vi "Send Message.vi"(6 "priority":i32, 8 "error in (no error)":errorcluster, 9 "timeout ms (-1)":i32=-1, 10 "Message":refnum<class "Message.lvclass">, 11 "Network Stream in":refnum<class "Network Stream.lvclass">) -> (0 "error out":errorcluster, 3 "Network Stream out":refnum<class "Network Stream.lvclass">)   [LabVIEW 2023, in "Network Stream.lvclass"]
uses:
  Network Stream.lvclass
  C:/Program Files/National Instruments/LabVIEW 2023/vi.lib/ni/Actors/Network Endpoint Actors/Abstract Classes/Message Stream/Message Stream.lvclass
  <vilib>/ActorFramework/Message/Message.lvclass
  <vilib>/ni/Actors/Network Endpoint Actors/Abstract Classes/Message Stream/Message Stream.lvclass/Message Stream.ctl
  Network Stream.lvclass/Network Stream.ctl
  <vilib>/ni/Actors/Network Endpoint Actors/Abstract Classes/Cipher/Cipher.lvclass
  <vilib>/ni/Actors/Network Endpoint Actors/Abstract Classes/Message Stream/Message Stream.lvclass
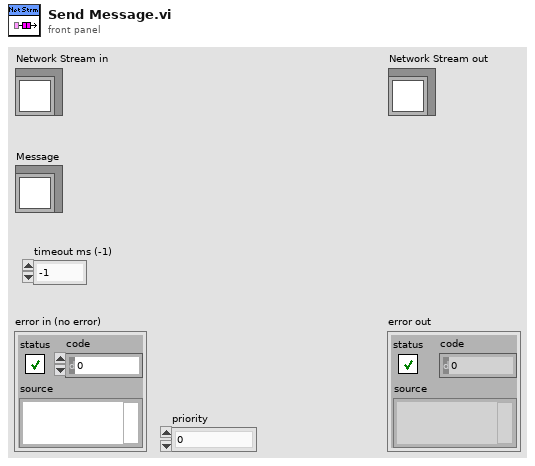
[diagram p1: front panel]
types:
  T1 = cluster{"Message":refnum<class "Message.lvclass">, "priority":i32}
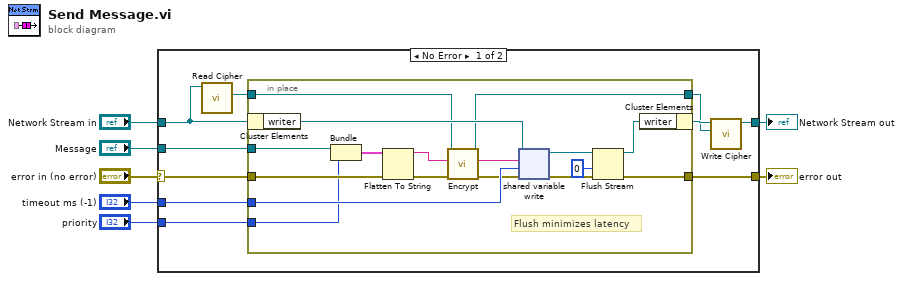
[diagram p0: block diagram]
diagram:
  n1 = case shown="No Error" "error in (no error)" {
    selector: "error in (no error)" -> [w17 w35]
    tunnel: "Network Stream in" -> [w10 w36]
    tunnel: [w16 w35] -> w5
    tunnel: [w11 w36] -> w4
    tunnel: "timeout ms (-1)" -> [w15 _]
    tunnel: "Message" -> [w14 _]
    tunnel: "priority" -> [w13 _]
    frame No Error {
      n2 = call <vilib>:"Read Cipher.vi"("Message Stream in"=w10) -> ("Cipher.lvclass"=w9:refnum<class "Cipher.lvclass">)  [unwired: 10 in]
      n3 = in-place {
        in-place-border: w17 -> [w33]
        in-place-border: [w21] -> w16
        in-place-border: w15 -> [w32]
        in-place-border: w14 -> [w31]
        in-place-border: w13 -> [w29]
        in-place-border: w9 -> [w24]
        in-place-border: [w23] -> w8
        # "Flush minimizes latency"
        n4 = in-place-cluster #1(w10) -> ("writer"=w34:refnum<k21>)
        n5 = Bundle("Message"=w31, "priority"=w29) -> (w30:T1)  [unwired: 1 in]
        n6 = Flatten To String(anything=w30, error in (no error)=w33) -> (data string=w26:string, error out=w28:errorcluster)  [unwired: 2 in, 1 out]
        n7 = call-dynamic "Encrypt.vi"("error in (no error)"=w28, "Plaintext"=w26, "Cipher in"=w24) -> ("error out"=w27:errorcluster, "Cyphertext"=w25:string, "Cipher out"=w23:refnum<class "Cipher.lvclass">)  [unwired: 6 in]
        n8 = shared-variable-write(w34, w27, w25, w32) -> (w19:refnum<k21>, w22:errorcluster)  [unwired: 1 out]
        n9 = Flush Stream(8:w22, 9:0 ("timeout in ms (-1)"), 11:w19) -> (0:w21:errorcluster, 3:w18:refnum<k21>)  [unwired: 1 in, 1 out]
        n10 = in-place-cluster #1("writer"=w18) -> (w12:refnum<class "Network Stream.lvclass">)
      }
      n11 = call <vilib>:"Write Cipher.vi"("Cipher"=w8, "Message Stream in"=w12) -> ("Message Stream out"=w11:refnum<class "Network Stream.lvclass">)  [unwired: 9 in]
    }
    frame Error {
    }
  }
  "error out" <- w5
  "Network Stream out" <- w4
